vi "Set Logging Base Path.vi"(8 "error in (no error)":errorcluster, 10 "Logging Base Path":path, 11 "Sensor in":refnum<class "Sensor.lvclass">) -> (0 "error out":errorcluster, 3 "Sensor out":refnum<class "Sensor.lvclass">)   [LabVIEW 2018, in "Sensor.lvlib" / "Sensor.lvclass"]
doc: "Updates the Base Path for the log file for the Sensor Actor. Deeper directories are composed of dates in the format: \n\nC:\\..\\YYYY\\MM\\DD"
uses:
  Sensor.lvclass
  Sensor.lvclass/Sensor.ctl
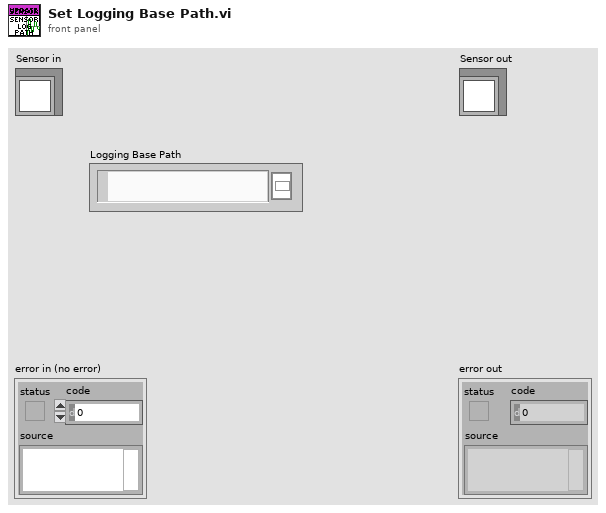
[diagram p1: front panel]
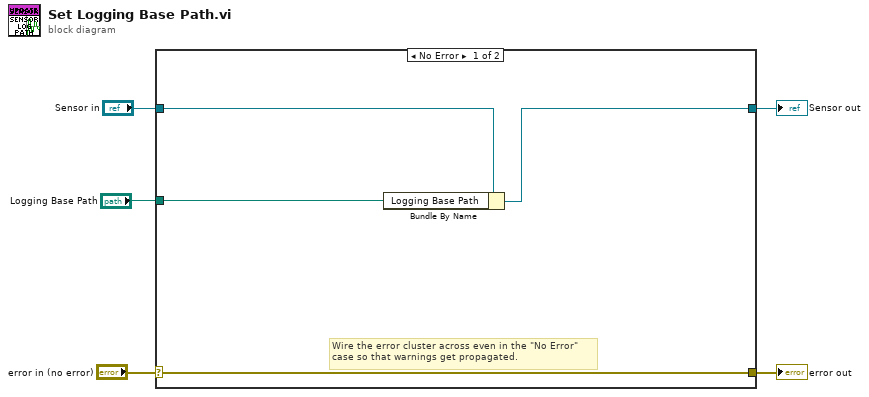
[diagram p0: block diagram]
diagram:
  n1 = case shown="No Error" "error in (no error)" {
    selector: "error in (no error)" -> [w9 w11]
    tunnel: [w9 w11] -> w4
    tunnel: [w7 w10] -> w2
    tunnel: "Sensor in" -> [w8 w10]
    tunnel: "Logging Base Path" -> [w6 _]
    frame No Error {
      # "Wire the error cluster across even in the \"No Error\"\ncase so that warnings get propagated."
      n2 = Bundle By Name(cluster=w8, "Logging Base Path"=w6) -> (w7:refnum<class "Sensor.lvclass">)
    }
    frame Error {
    }
  }
  "error out" <- w4
  "Sensor out" <- w2
